vi "Write.vi"(10 "Path Array":path[](array[path]), 11 "Path Array in":refnum<class "Path Array.lvclass">) -> (3 "Path Array out":refnum<class "Path Array.lvclass">)   [LabVIEW 2020, in "Data.lvlib" / "Path Array.lvclass"]
doc: "Write String Array."
uses:
  Path Array.lvclass
  Path Array.lvclass/Path Array.ctl
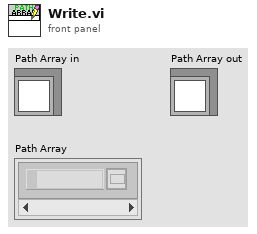
[diagram p1: front panel]
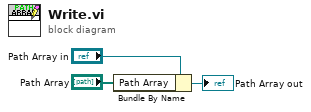
[diagram p0: block diagram]
diagram:
  n1 = Bundle By Name(cluster="Path Array in", "Path Array"="Path Array") -> (→"Path Array out":refnum<class "Path Array.lvclass">)
